vi "DANTE init & config_test.vi"(8 "Boards to configure":u8(slide) scale=0.0..8.0, 10 "Number of boards in chain":u8(slide)=1 scale=1.0..8.0, 11 "IP Address":string="10.96.0.110") -> (0 "x != 0?":bool, 1 "DANTE loaded":bool, 2 "IP added":bool, 3 "Library Initialized":bool, 5 "identifier out":string)   [LabVIEW 2015]
uses:
  libs/Initialization.ctl
  Scanning Software_Demokritos_2015_v7/libs/XGL_DPP.lvlib
panel:
  out "initialized array":u32[](array[numeric])
  out "data out":u32[](array[numeric])
  out "Error code":i32
  in  "Acquisition time [s]":dbl=10.0 min=1.0 max=1000.0
  out "State":T1
  in  "DPP Configuration 2":T2={"reset_recovery_time"=300, "edge_peaking_time"=4, "flat_top"=7, "peaking_time"=32, "gain"=1.0, "max_risetime"=0.0, "fast_filter_thr"=45, "zero_peak_freq"=1.0, "inverted_input"=0, "base_offset"=0, "reset_threshold"=1000, "overflow_recovery"=0, "tail_coefficient"=0.0, "energy_filter_thr"=23, "energy_baseline_thr"=23, "max_peaking_time"=35, "edge_flat_top"=1, "time_constant"=0.0, "baseline_samples"=64, "other_param"=0}
  in  "stop":bool
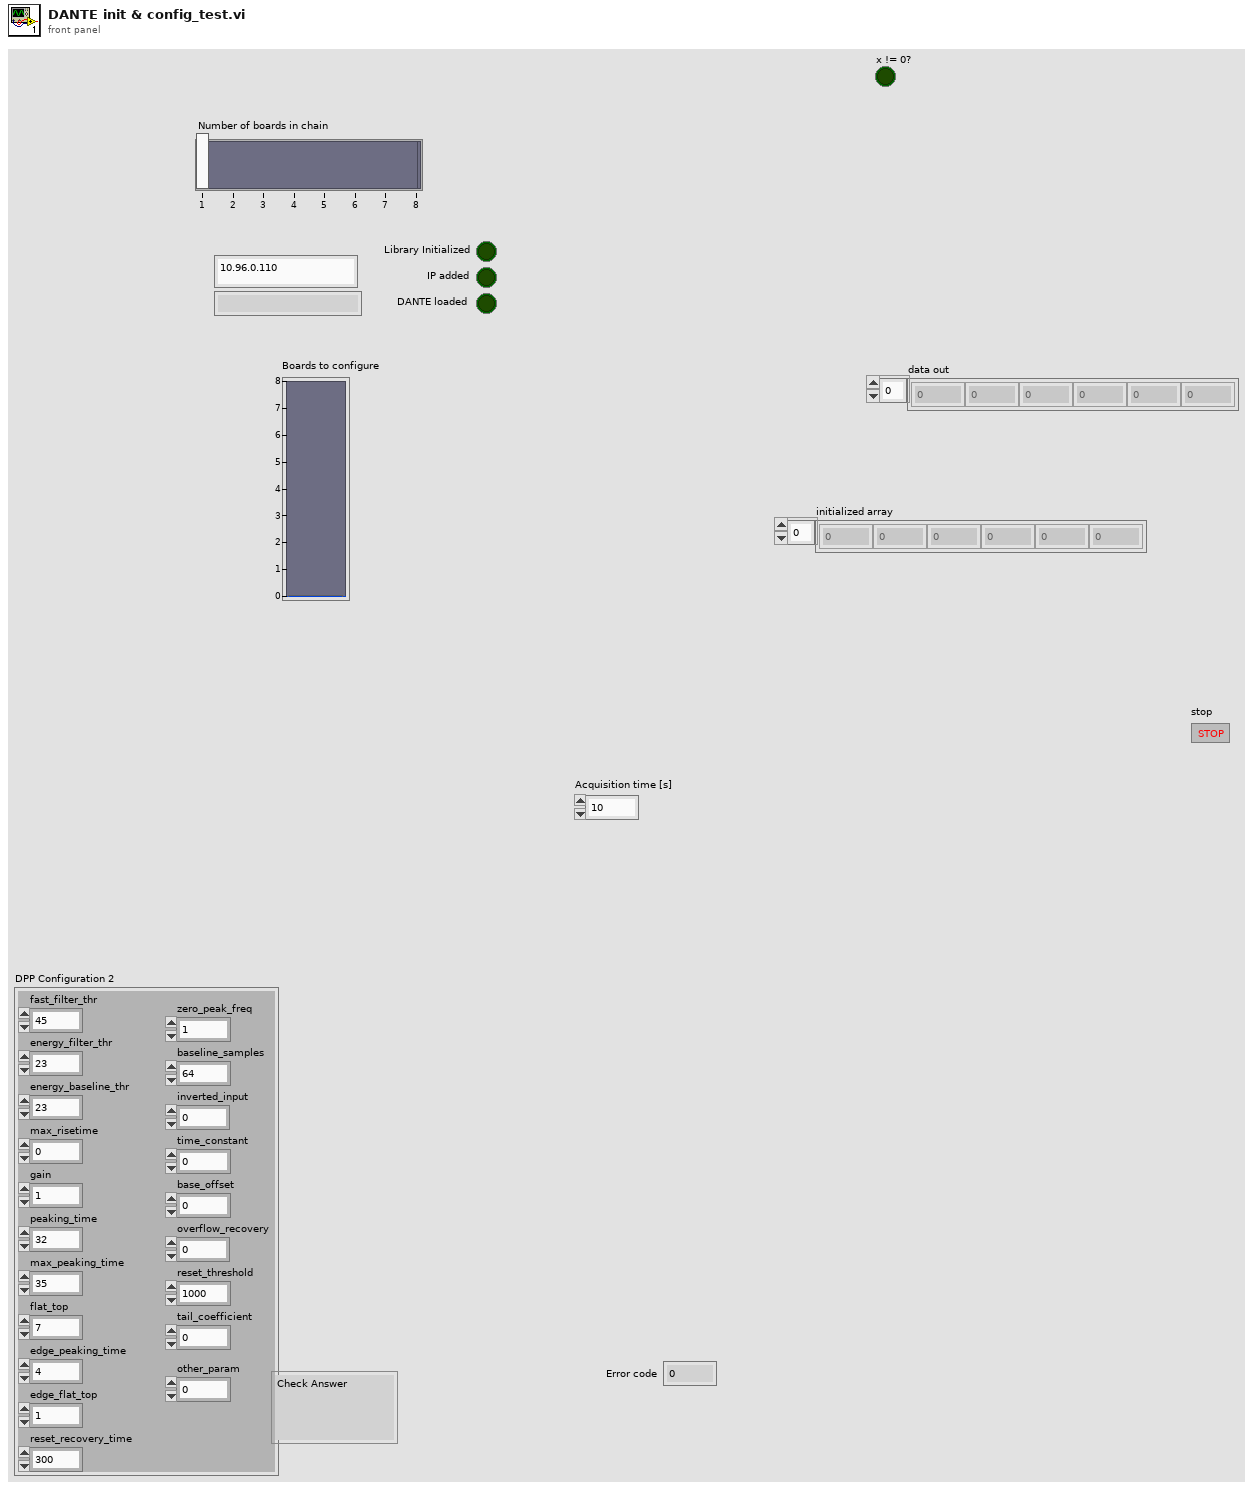
[diagram p1: front panel]
types:
  T1 = typedef "Initialization.ctl" = enum16{"Check Answer", "Configuring", "Wait Answer"}
  T2 = cluster{"reset_recovery_time":u32, "edge_peaking_time":u32, "flat_top":u32, "peaking_time":u32, "gain":dbl, "max_risetime":dbl, "fast_filter_thr":u32, "zero_peak_freq":dbl, "inverted_input":u8, "base_offset":u32, "reset_threshold":u32, "overflow_recovery":u32, "tail_coefficient":dbl, "energy_filter_thr":u32, "energy_baseline_thr":u32, "max_peaking_time":u32, "edge_flat_top":u32, "time_constant":dbl, "baseline_samples":u32, "other_param":u32}
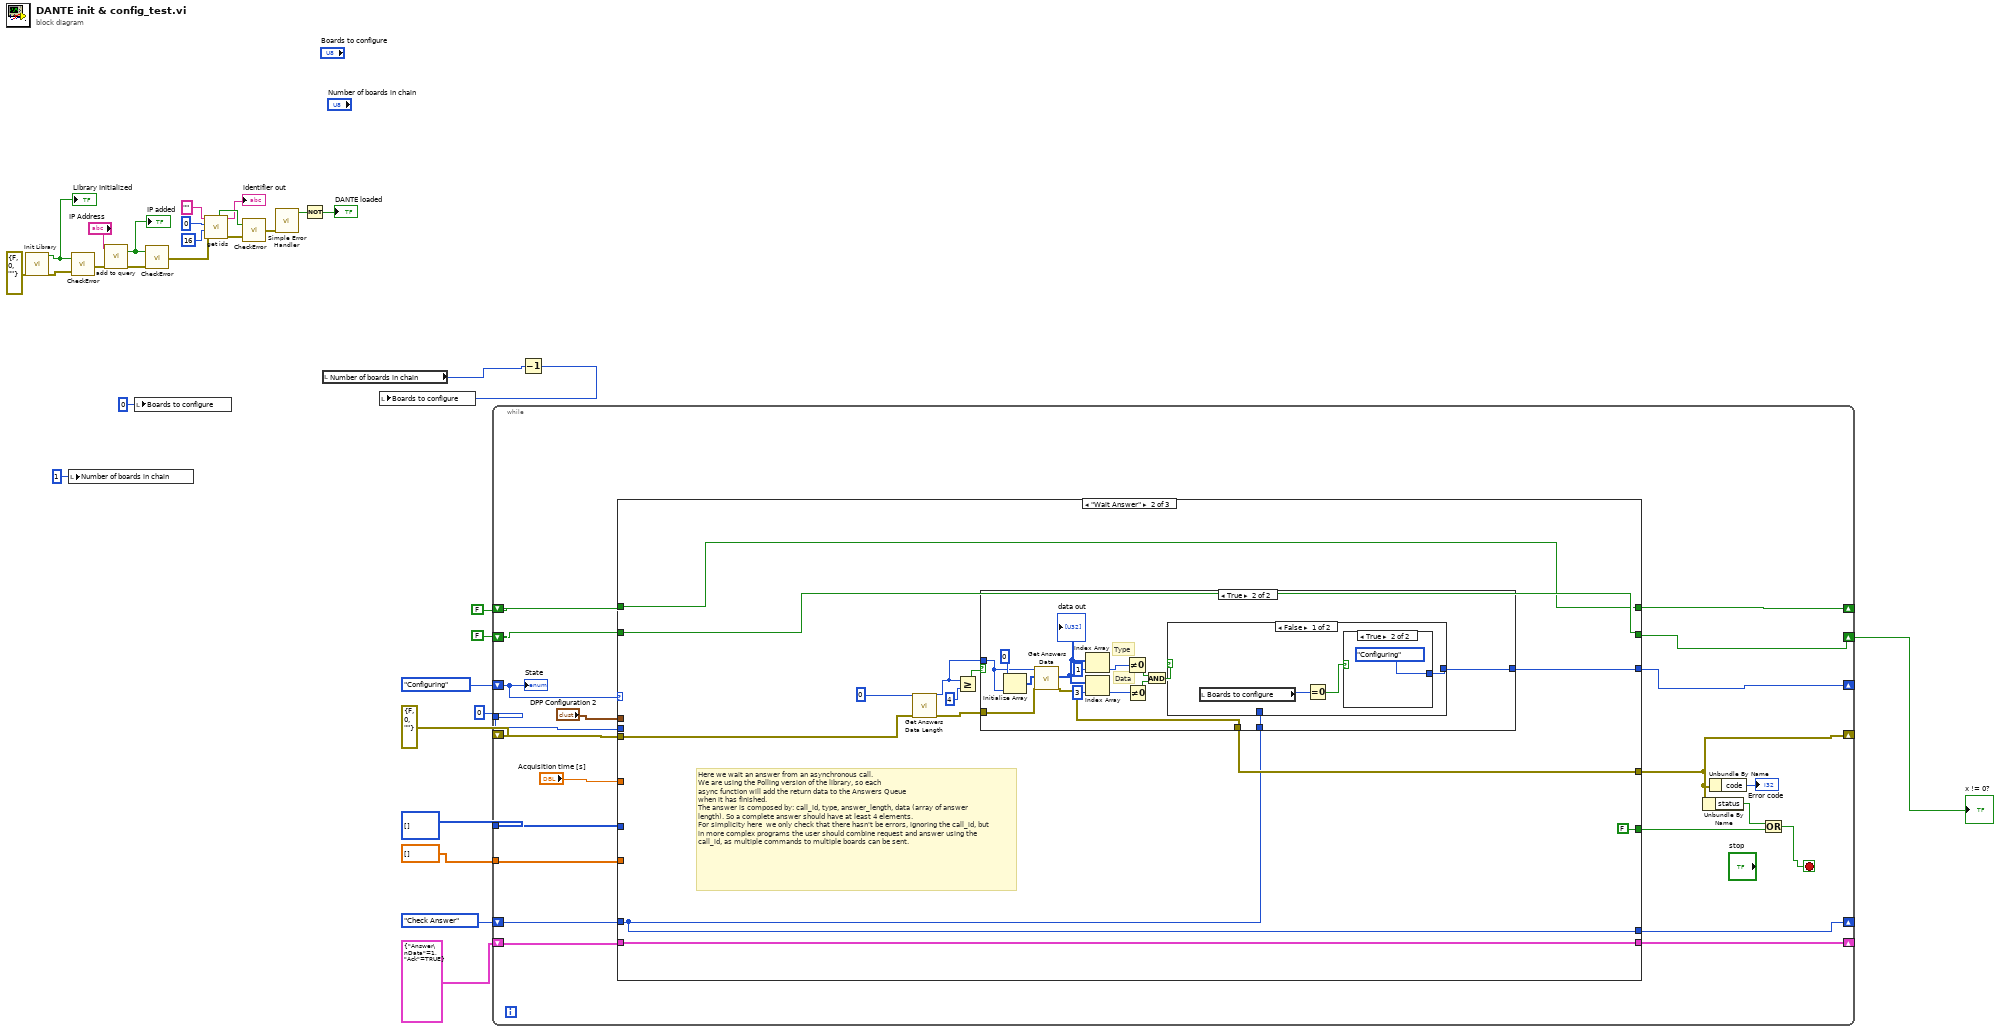
[diagram p0: block diagram]
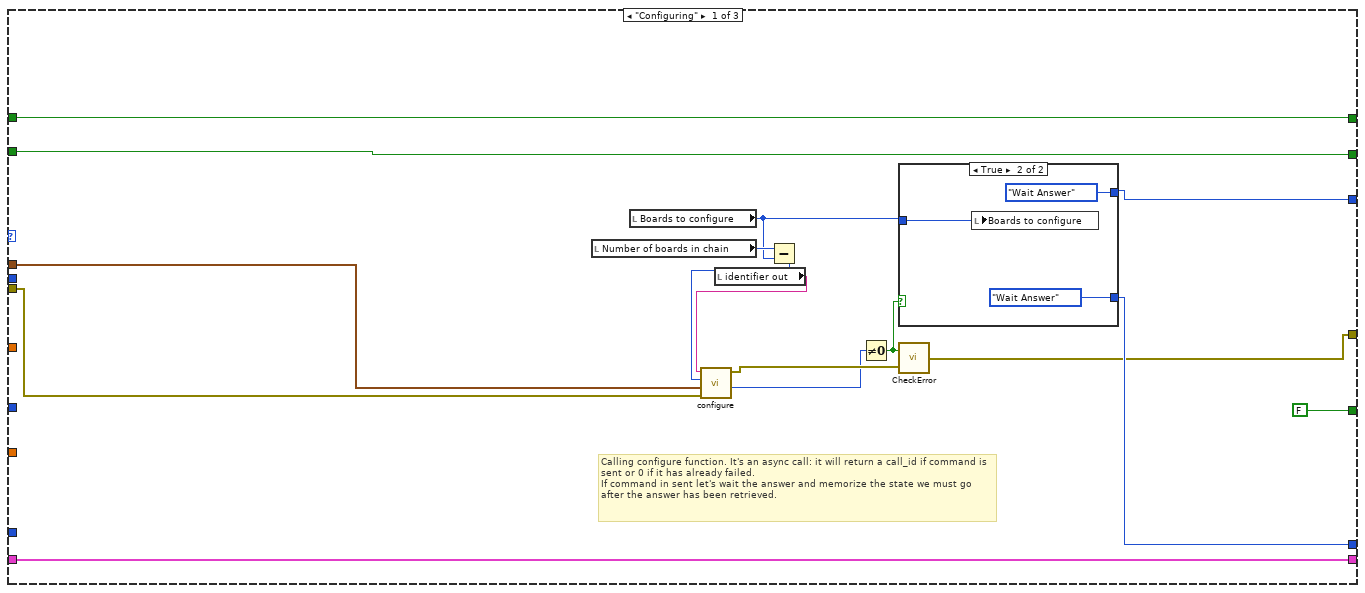
[diagram p2: hidden frame]
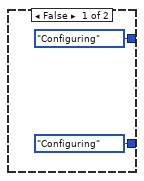
[diagram p3: hidden frame]
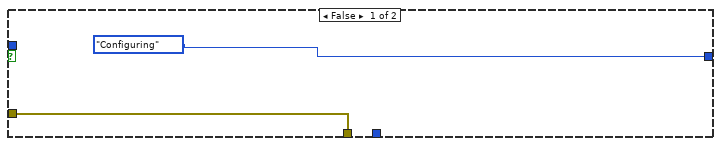
[diagram p4: hidden frame]
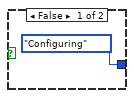
[diagram p5: hidden frame]
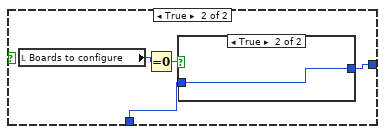
[diagram p6: hidden frame]
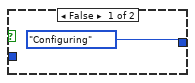
[diagram p7: hidden frame]
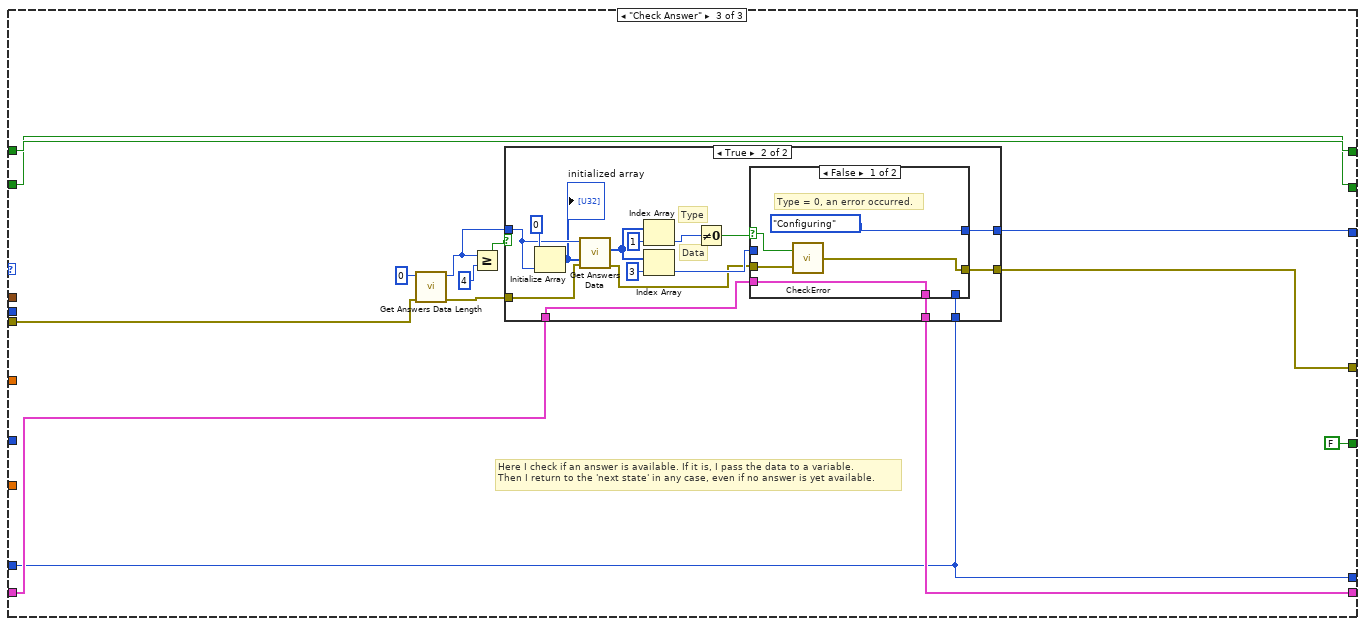
[diagram p8: hidden frame]
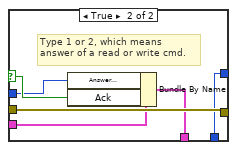
[diagram p10: hidden frame]
diagram:
  n1 = call "Init Library.vi"("error in (no error)"=errorcluster {"status"=FALSE, "code"=0, "source"=""}) -> ("error out"=w18:errorcluster, "function return"=w19:bool)  [unwired: 9 in]
  "Library Initialized" <- w19
  n2 = local write "Number of boards in chain"(u8 1 ("Number of boards in chain")) -> ()
  n3 = call "CheckError.vi"("error in (no error)"=w18, "ret_val"=w19) -> ("error out"=w20:errorcluster)
  n4 = call "add to query.vi"("error in (no error)"=w20, "address"="IP Address") -> ("error out"=w22:errorcluster, "function return"=w23:bool)  [unwired: 7 in, 1 out]
  "IP added" <- w23
  n5 = local write "Boards to configure"(u8 0 ("Boards to configure")) -> ()
  n6 = call "CheckError.vi"("error in (no error)"=w22, "ret_val"=w23) -> ("error out"=w28:errorcluster)
  n7 = call "get ids.vi"("error in (no error)"=w28, "id_size"=u32 16 ("char_size"), "nb"=u32 0, "identifier"="") -> ("error out"=w15:errorcluster, "identifier out"=→"identifier out":string, "function return"=w25:bool)  [unwired: 3 in, 2 out]
  n8 = call "CheckError.vi"("error in (no error)"=w15, "ret_val"=w25) -> ("error out"=w29:errorcluster)
  n9 = call <vilib>:"Simple Error Handler.vi"("error in (no error)"=w29) -> ("error?"=w30:bool)  [unwired: 4 in, 4 out]
  n10 = Not(x=w30) -> (.not. x?=→"DANTE loaded":bool)
  n11 = local read "Number of boards in chain"() -> (w2:u8)
  n12 = while {
    shift-right: [w50] -> _
    shift-left: errorcluster {"status"=FALSE, "code"=0, "source"=""} ("error in (no error)") -> [w52]
    shift-right: [w39] -> _
    shift-left: Initialization."Configuring" ("State") -> [w36]
    shift-right: [w45] -> _
    shift-left: FALSE -> [w46]
    shift-right: [w43] -> w3
    shift-left: FALSE -> [w44]
    tunnel: u16 0 ("Board") -> [w42]
    shift-right: [w41] -> _
    shift-left: Initialization."Check Answer" ("State") -> [w40]
    shift-right: [w37] -> _
    shift-left: cluster{"Answer\nData":i32, "Ack":bool} {"Answer\nData"=1, "Ack"=TRUE} -> [w38]
    tunnel: dbl[] [] ("Y") -> [w35]
    tunnel: u16[][] [] ("element") -> [w34]
    stop <- w32 stop-if-true
    n13 = case shown="\"Wait Answer\"" w36 {
      tunnel: w52 -> [w57 w86 w122]
      tunnel: [w63 w80 w121] -> w50
      tunnel: [w64 w77 w120] -> w39
      tunnel: "Acquisition time [s]" -> [_ _ _]
      tunnel: [FALSE ("y") FALSE ("y") FALSE ("y")] -> w47
      tunnel: [w67 w74 w116] -> w45
      tunnel: w46 -> [w67 w74 w116]
      tunnel: [w66 w78 w115] -> w43
      tunnel: w44 -> [w66 w78 w115]
      tunnel: w42 -> [_ _ _]
      tunnel: [w65 w76 w117] -> w41
      tunnel: w40 -> [_ w76 w117]
      tunnel: "DPP Configuration 2" -> [w58 _ _]
      tunnel: w38 -> [w62 w75 w119]
      tunnel: [w62 w75 w118] -> w37
      tunnel: w34 -> [_ _ _]
      tunnel: w35 -> [_ _ _]
      frame "Configuring" {
        # "Calling configure function. It's an async call: it will return a call_id if command is sent or 0 if it has already failed.\nIf command in sent let's wait the answer and memorize the state we must go after the answer has been retrieved."
        n14 = local read "Number of boards in chain"() -> (w60:u8)
        n15 = local read "Boards to configure"() -> (w59:u8)
        n16 = local read "identifier out"() -> (w56:string)
        n17 = Subtract(x=w60, y=w59) -> (x-y=w55:u8)
        n18 = call "configure.vi"("error in (no error)"=w57, "DPP Configuration"=w58, "Board"=w55, "identifier"=w56) -> ("function return"=w53:u32, "error out"=w54:errorcluster)  [unwired: 2 in]
        n19 = Not Equal To 0?(x=w53) -> (x != 0?=w61:bool)
        n20 = case shown="True" w61 {
          tunnel: [Initialization."Configuring" ("State") Initialization."Wait Answer" ("State")] -> w64
          tunnel: [Initialization."Configuring" ("State") Initialization."Wait Answer" ("State")] -> w65
          tunnel: w59 -> [_ w71]
          frame False {
          }
          frame True {
            n21 = local write "Boards to configure"(w71) -> ()
          }
        }
        n22 = call "CheckError.vi"("error in (no error)"=w54, "ret_val"=w61) -> ("error out"=w63:errorcluster)
      }
      frame "Wait Answer" {
        # "Here we wait an answer from an asynchronous call.\nWe are using the Polling version of the library, so each\nasync function will add the return data to the Answers Queue\nwhen it has finished.\nThe answer is composed by: call_id, type, answer_length, data (array of answer length). So a complete answer should have at least 4 elements.\nFor simplicity here  we only check that there hasn't be errors, ignoring the call_id, but in more complex programs the user should combine request and answer using the call_id, as multiple commands to multiple boards can be sent."
        n23 = call "Get Answers Data Length.vi"("error in (no error)"=w86, "length"=u32 0) -> ("error out"=w82:errorcluster, "length out"=w81:u32)  [unwired: 7 in, 1 out]
        n24 = Greater Or Equal?(x=w81, y=u32 4) -> (x >= y?=w83:bool)
        n25 = case shown="True" w83 {
          tunnel: w82 -> [w88 w91]
          tunnel: w81 -> [_ w93]
          tunnel: w76 -> [_ w95]
          tunnel: [w88 w90] -> w80
          tunnel: [Initialization."Configuring" ("State") w94] -> w77
          frame False {
          }
          frame True {
            # "Data"
            # "Type"
            n26 = Initialize Array(u32 0 ("y"), w93) -> (w92:u32[])
            n27 = call "Get Answers Data.vi"("error in (no error)"=w91, "data"=w92, "length"=w93) -> ("error out"=w90:errorcluster, "data out"=w89:u32[])  [unwired: 4 in, 1 out]
            "data out" <- w89
            n28 = Index Array(array=w89, index=1) -> (element=w99:u32)
            n29 = Index Array(array=w89, index=3) -> (element=w100:u32)
            n30 = Not Equal To 0?(x=w99) -> (x != 0?=w97:bool)
            n31 = Not Equal To 0?(x=w100) -> (x != 0?=w98:bool)
            n32 = And(x=w97, y=w98) -> (x .and. y?=w96:bool)
            n33 = case shown="False" w96 {
              tunnel: w95 -> [_ w109]
              tunnel: [w106 w110] -> w94
              frame False {
                n34 = local read "Boards to configure"() -> (w105:u8)
                n35 = Equal To 0?(x=w105) -> (x = 0?=w104:bool)
                n36 = case shown="True" w104 {
                  tunnel: [Initialization."Configuring" ("State") Initialization."Configuring" ("State")] -> w106
                  frame False {
                  }
                  frame True {
                  }
                }
              }
              frame True {
                n37 = local read "Boards to configure"() -> (w112:u8)
                n38 = Equal To 0?(x=w112) -> (x = 0?=w111:bool)
                n39 = case shown="True" w111 {
                  tunnel: [Initialization."Configuring" ("State") w114] -> w110
                  tunnel: w109 -> [_ w114]
                  frame False {
                  }
                  frame True {
                  }
                }
              }
            }
          }
        }
      }
      frame "Check Answer" {
        # "Here I check if an answer is available. If it is, I pass the data to a variable.\nThen I return to the 'next state' in any case, even if no answer is yet available."
        n40 = call "Get Answers Data Length.vi"("error in (no error)"=w122, "length"=u32 0) -> ("error out"=w124:errorcluster, "length out"=w123:u32)  [unwired: 7 in, 1 out]
        n41 = Greater Or Equal?(x=w123, y=u32 4) -> (x >= y?=w125:bool)
        n42 = case shown="True" w125 {
          tunnel: w124 -> [w131 w136]
          tunnel: w123 -> [_ w134]
          tunnel: [w131 w142] -> w121
          tunnel: [w130 w141] -> w120
          tunnel: w117 -> [w130 w140]
          tunnel: w119 -> [w129 w138]
          tunnel: [w129 w139] -> w118
          frame False {
            # "Do not update answer data."
          }
          frame True {
            # "Data"
            # "Type"
            n43 = Initialize Array(u32 0 ("y"), w134) -> (w132:u32[])
            "initialized array" <- w132
            n44 = call "Get Answers Data.vi"("error in (no error)"=w136, "data"=w132, "length"=w134) -> ("error out"=w135:errorcluster, "data out"=w133:u32[])  [unwired: 4 in, 1 out]
            n45 = Index Array(array=w133, index=1) -> (element=w144:u32)
            n46 = Index Array(array=w133, index=3) -> (element=w137:u32)
            n47 = Not Equal To 0?(x=w144) -> (x != 0?=w143:bool)
            n48 = case shown="False" w143 {
              selector: w143 -> [w152 w154]
              tunnel: w135 -> [w151 w158]
              tunnel: [w150 w158] -> w142
              tunnel: [Initialization."Configuring" ("State") w157] -> w141
              tunnel: w140 -> [_ w157]
              tunnel: [w149 w155] -> w139
              tunnel: w138 -> [w149 w156]
              tunnel: w137 -> [_ w153]
              frame False {
                # "Type = 0, an error occurred."
                n49 = call "CheckError.vi"("error in (no error)"=w151, "ret_val"=w152) -> ("error out"=w150:errorcluster)
              }
              frame True {
                # "Type 1 or 2, which means\nanswer of a read or write cmd."
                n50 = Bundle By Name(cluster=w156, "Answer\nData"=w153, "Ack"=w154) -> (w155:cluster{"Answer\nData":i32, "Ack":bool})
              }
            }
          }
        }
      }
    }
    n51 = Unbundle By Name(w50) -> ("status"=w48:bool)
    n52 = Unbundle By Name(w50) -> ("code"=→"Error code":i32)
    n53 = Or(x=w48, y=w47) -> (x .or. y?=w32:bool)
    "State" <- w36
  }
  "x != 0?" <- w3
  n54 = Decrement(x=w2) -> (x-1=w1:u8)
  n55 = local write "Boards to configure"(w1) -> ()
